vi "IsoSPI Spying Tool data interpretation (1).vi"(9 "nbmodule":i32=8, 11 "String from arduino":string) -> (2 "Vcell":dbl[][](array[numeric]), 3 "TCELL":dbl[][](array[numeric]))   [LabVIEW 2020]
panel:
  out "Numérique":i32
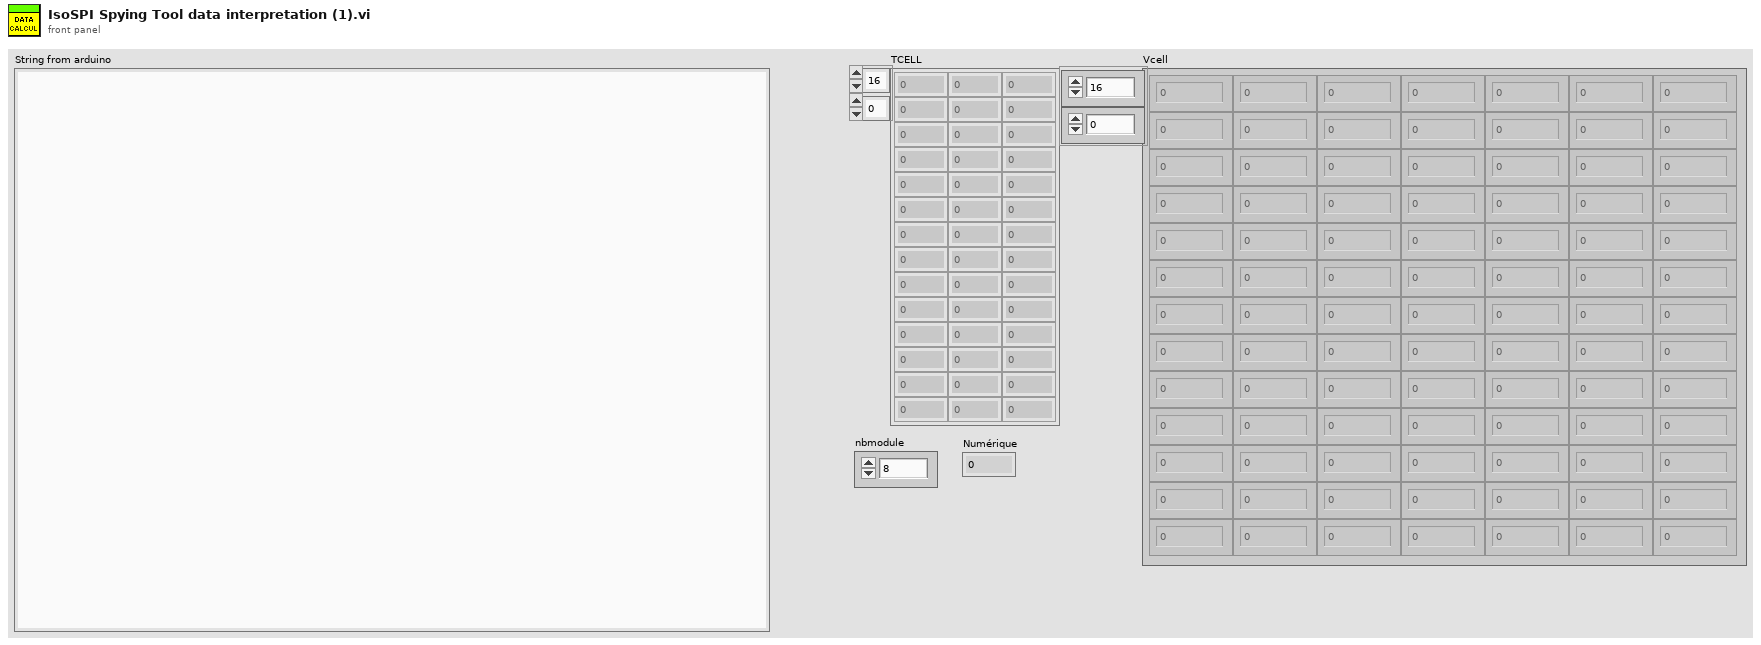
[diagram p1: front panel]
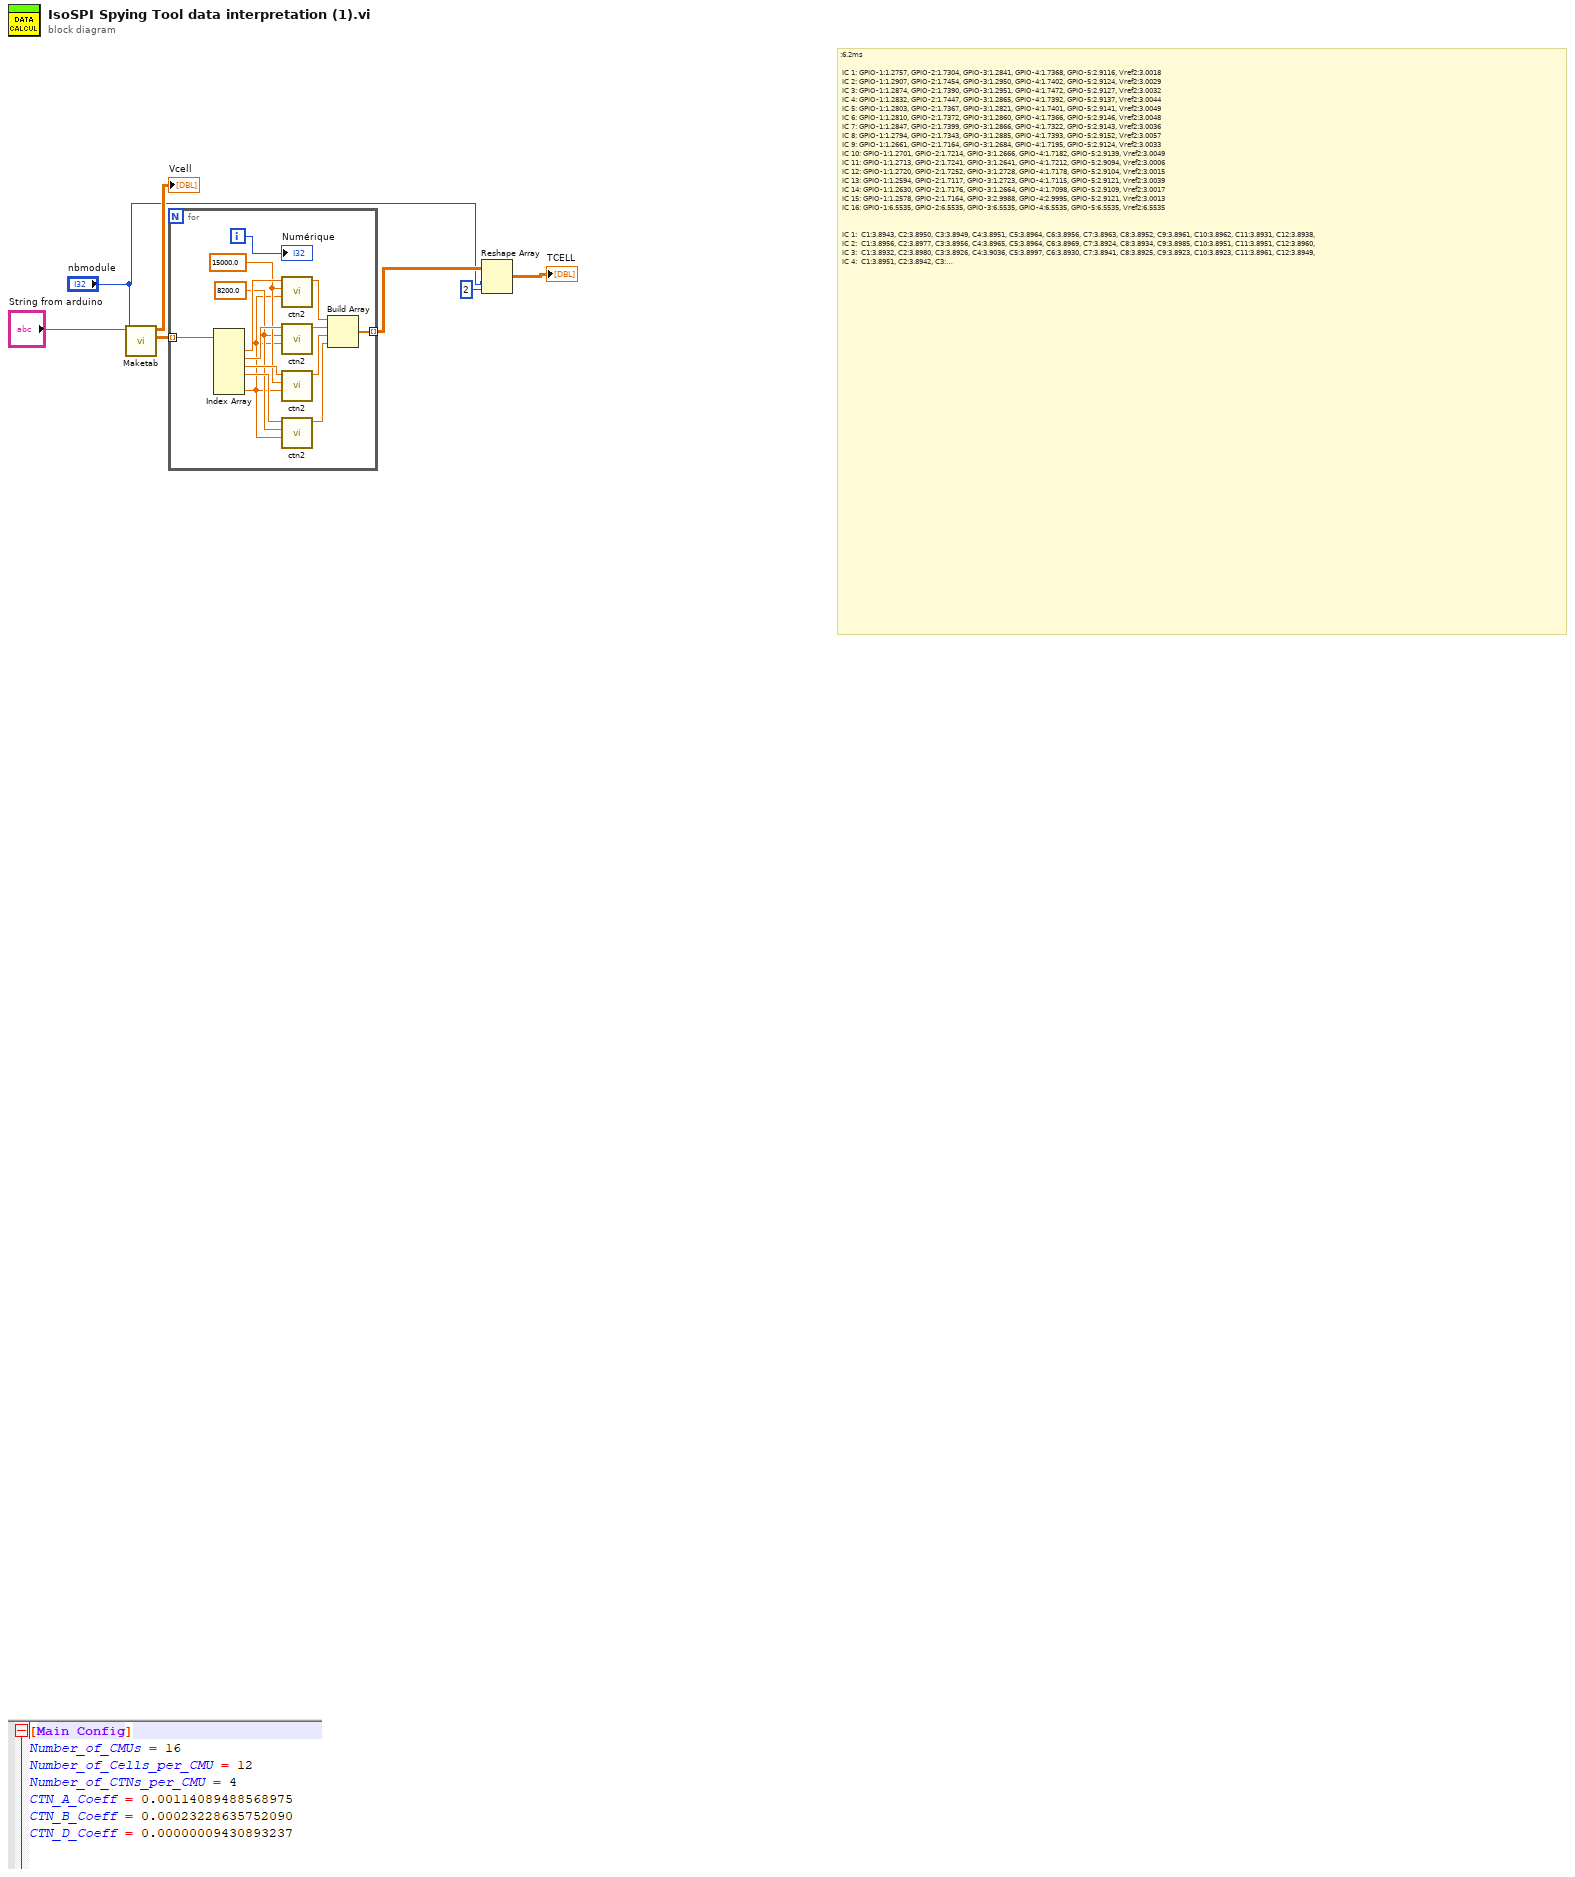
[diagram p0: block diagram]
diagram:
  # ":6.2ms \n\n IC 1: GPIO-1:1.2757, GPIO-2:1.7304, GPIO-3:1.2841, GPIO-4:1.7368, GPIO-5:2.9116, Vref2:3.0018\n IC 2: GPIO-1:1.2907, GPIO-2:1.7454, GPIO-3:1.2950, GPIO-4:1.7402, GPIO-5:2.9124, Vref2:3.0029\n IC 3: GPIO-1:1.2874, GPIO-2:1.7390, GPIO-3:1.2951, GPIO-4:1.7472, GPIO-5:2.9127, Vref2:3.0032\n IC 4: GPIO-1:1.2832, GPIO-2:1.7447, GPIO-3:1.2865, GPIO-4:1.7392, GPIO-5:2.9137, Vref2:3.0044\n IC 5: GPIO-1:1.2803, GPIO-2:1.7367, GPIO-3:1.2821, GPIO-4:1.7401, GPIO-5:2.9141, Vref2:3.0049\n IC 6: GPIO-1:1.2810, GPIO-2:1.7372, GPIO-3:1.2860, GPIO-4:1.7366, GPIO-5:2.9146, Vref2:3.0048\n IC 7: GPIO-1:1.2847, GPIO-2:1.7399, GPIO-3:1.2866, GPIO-4:1.7322, GPIO-5:2.9143, Vref2:3.0036\n IC 8: GPIO-1:1.2794, GPIO-2:1.7343, GPIO-3:1.2885, GPIO-4:1.7393, GPIO-5:2.9152, Vref2:3.0057\n IC 9: GPIO-1:1.2661, GPIO-2:1.7164, GPIO-3:1.2684, GPIO-4:1.7195, GPIO-5:2.9124, Vref2:3.0033\n IC 10: GPIO-1:1.2701, GPIO-2:1.7214, GPIO-3:1.2666, GPIO-4:1.7182, GPIO-5:2.9139, Vref2:3.0049\n IC 11: GPIO-1:1.2713, GPIO-2:1.7241, GPIO-3:1.2641, GPIO-4:1.7212, GPIO-5:2.9094, Vref2:3.0006\n IC 12: GPIO-1:1.2720, GPIO-2:1.7252, GPIO-3:1.2728, GPIO-4:1.7178, GPIO-5:2.9104, Vref2:3.0015\n IC 13: GPIO-1:1.2594, GPIO-2:1.7117, GPIO-3:1.2723, GPIO-4:1.7115, GPIO-5:2.9121, Vref2:3.0039\n IC 14: GPIO-1:1.2630, GPIO-2:1.7176, GPIO-3:1.2664, GPIO-4:1.7098, GPIO-5:2.9109, Vref2:3.0017\n IC 15: GPIO-1:1.2578, GPIO-2:1.7164, GPIO-3:2.9988, GPIO-4:2.9995, GPIO-5:2.9121, Vref2:3.0013\n IC 16: GPIO-1:6.5535, GPIO-2:6.5535, GPIO-3:6.5535, GPIO-4:6.5535, GPIO-5:6.5535, Vref2:6.5535\n\n\n IC 1:  C1:3.8943, C2:3.8950, C3:3.8949, C4:3.8951, C5:3.8964, C6:3.8956, C7:3.8963, C8:3.8952, C9:3.8961, C10:3.8962, C11:3.8931, C12:3.8938,\n IC 2:  C1:3.8956, C2:3.8977, C3:3.8956, C4:3.8965, C5:3.8964, C6:3.8969, C7:3.8924, C8:3.8934, C9:3.8985, C10:3.8951, C11:3.8951, C12:3.8960,\n IC 3:  C1:3.8932, C2:3.8980, C3:3.8926, C4:3.9036, C5:3.8997, C6:3.8930, C7:3.8941, C8:3.8925, C9:3.8923, C10:3.8923, C11:3.8961, C12:3.8949,\n IC 4:  C1:3.8951, C2:3.8942, C3:3.8941, C4:3.8960, C5:3.8947, C6:3.8913, C7:3.8944, C8:3.8953, C9:3.8961, C10:3.8916, C11:3.8926, C12:3.8935,\n IC 5:  C1:3.8971, C2:3.8957, C3:3.8947, C4:3.8935, C5:3.8936, C6:3.8945, C7:3.8967, C8:3.8957, C9:3.8931, C10:3.8944, C11:3.8915, C12:3.8947,\n IC 6:  C1:3.8948, C2:3.8933, C3:3.8951, C4:3.8939, C5:3.8964, C6:3.8926, C7:3.8950, C8:3.8936, C9:3.8921, C10:3.8948, C11:3.8970, C12:3.8943,\n IC 7:  C1:3.8961, C2:3.9015, C3:3.8999, C4:3.8979, C5:3.8988, C6:3.9047, C7:3.8957, C8:3.8934, C9:3.8937, C10:3.8960, C11:3.8923, C12:3.8923,\n IC 8:  C1:3.8939, C2:3.8939, C3:3.8937, C4:3.8928, C5:3.8950, C6:3.8954, C7:3.8930, C8:3.8948, C9:3.8937, C10:3.8942, C11:3.8963, C12:3.8968,\n IC 9:  C1:3.8957, C2:3.8958, C3:3.8942, C4:3.8954, C5:3.8955, C6:3.8938, C7:3.8941, C8:3.8940, C9:3.8940, C10:3.8943, C11:3.8918, C12:3.8950,\n IC 10:  C1:3.8960, C2:3.8925, C3:3.8922, C4:3.8923, C5:3.8906, C6:3.8949, C7:3.8938, C8:3.8937, C9:3.8937, C10:3.8930, C11:3.8910, C12:3.8932,\n IC 11:  C1:3.8980, C2:3.8943, C3:3.8965, C4:3.8933, C5:3.8944, C6:3.8935, C7:3.8952, C8:3.8928, C9:3.8924, C10:3.8943, C11:3.8928, C12:3.8935,\n IC 12:  C1:3.8972, C2:3.8956, C3:3.8958, C4:3.8950, C5:3.8952, C6:3.8944, C7:3.8963, C8:3.8964, C9:3.8945, C10:3.8941, C11:3.8939, C12:3.8943,\n IC 13:  C1:3.8937, C2:3.8941, C3:3.8960, C4:3.8961, C5:3.8971, C6:3.8978, C7:3.9043, C8:3.9041, C9:3.8952, C10:3.8956, C11:3.8947, C12:3.8904,\n IC 14:  C1:3.8969, C2:3.8921, C3:3.8978, C4:3.8939, C5:3.8961, C6:3.8947, C7:3.8964, C8:3.8941, C9:3.8955, C10:3.8948, C11:3.8955, C12:3.8956,\n IC 15:  C1:3.8938, C2:3.8952, C3:3.8943, C4:0.0000, C5:0.0000, C6:0.0000, C7:3.8954, C8:3.8949, C9:3.8944, C10:0.0000, C11:0.0000, C12:0.0000,\n IC 16:  C1:6.5535, C2:6.5535, C3:6.5535, C4:6.5535, C5:6.5535, C6:6.5535, C7:6.5535, C8:6.5535, C9:6.5535, C10:6.5535, C11:6.5535, C12:6.5535,"
  n1 = call "Maketab.vi"("nbmodule"="nbmodule", "Chaîne"="String from arduino") -> ("Tcell"=w6:dbl[][], "Vcell"=→"Vcell":dbl[][])  [unwired: 7 in, 1 out]
  n2 = for {
    tunnel: w6 -> [w20] mode=indexing
    tunnel: [w8] -> w4 mode=indexing
    i -> [w21]
    w14 = 8200.0 ("x")
    w15 = 15000.0 ("x")
    n3 = Index Array(array=w20) -> (element #1=w19:dbl, element #2=w18:dbl, element #3=w16:dbl, element #4=w17:dbl, element #6=w13:dbl)  [unwired: 6 in, 1 out]
    n4 = call "ctn2.vi"("Numérique 2"=w13, "x"=w15, "Numérique"=w19) -> ("Numérique 3"=w12:dbl)  [unwired: 8 in]
    n5 = call "ctn2.vi"("Numérique 2"=w13, "x"=w14, "Numérique"=w18) -> ("Numérique 3"=w11:dbl)  [unwired: 8 in]
    n6 = call "ctn2.vi"("Numérique 2"=w13, "x"=w15, "Numérique"=w16) -> ("Numérique 3"=w10:dbl)  [unwired: 8 in]
    n7 = call "ctn2.vi"("Numérique 2"=w13, "x"=w14, "Numérique"=w17) -> ("Numérique 3"=w9:dbl)  [unwired: 8 in]
    n8 = Build Array(w12, w11, w10, w9) -> (w8:dbl[])
    "Numérique" <- w21
  }
  n9 = Reshape Array(w4, "nbmodule", 2 ("taille de la dimension")) -> (→"TCELL":dbl[][])
